vi "Publish Image.vi"(8 "error in (no error)":errorcluster, 9 "Buffer Number":u32, 10 "Image":T1, 11 "Camera in":refnum<class "Camera Actor.lvclass">) -> (0 "error out":errorcluster, 3 "Camera out":refnum<class "Camera Actor.lvclass">)   [LabVIEW 2020, in "Camera Actor.lvlib" / "Camera Actor.lvclass"]
uses:
  Camera Actor.lvclass
  <vilib>/vision/Image Controls.llb/IMAQ Image.ctl
  Camera Actor.lvclass/Camera Actor.ctl
  Camera Actor Messages/New Image Msg/New Image Msg.lvclass/New Image Msg.ctl
  <vilib>/ActorFramework/Message Enqueuer/Message Enqueuer.lvclass/Message Enqueuer.ctl
  <vilib>/ActorFramework/Message Enqueuer/Enqueue.vi
  Camera Actor Messages/New Image Msg/New Image Msg.lvclass
  C:/Program Files (x86)/National Instruments/LabVIEW 2020/vi.lib/ActorFramework/Message/Message.lvclass
  <vilib>/ActorFramework/Message Priority Queue/Priority Enqueue.vi
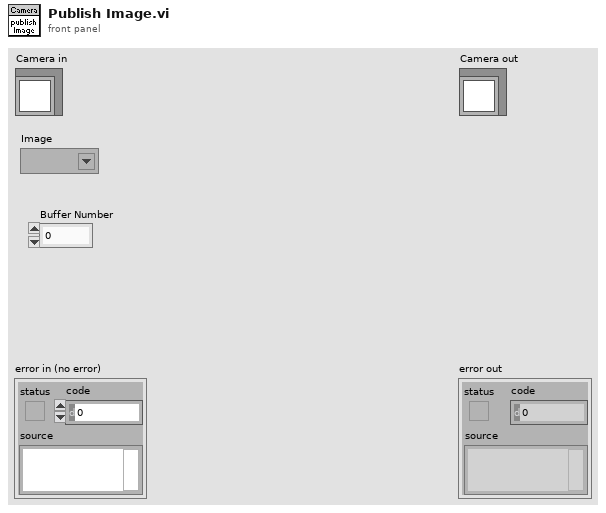
[diagram p1: front panel]
types:
  T1 = typedef "IMAQ Image.ctl" = refnum<image>
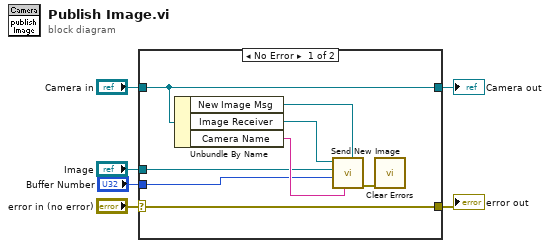
[diagram p0: block diagram]
diagram:
  n1 = case shown="No Error" "error in (no error)" {
    selector: "error in (no error)" -> [w13 w16]
    tunnel: [w13 w16] -> w5
    tunnel: [w12 w15] -> w3
    tunnel: "Camera in" -> [w12 w15]
    tunnel: "Image" -> [w10 _]
    tunnel: "Buffer Number" -> [w9 _]
    frame No Error {
      n2 = Unbundle By Name(w12) -> ("New Image Msg"=w8:refnum<class "New Image Msg.lvclass">, "Image Receiver"=w7:refnum<class "Message Enqueuer.lvclass">, "Camera Name"=w14:string)
      n3 = call "Send New Image.vi"("Message Type"=w8, "Camera"=w14, "Buffer Number"=w9, "Image"=w10, "Message Enqueuer"=w7) -> ("error out"=w11:errorcluster)  [unwired: 5 in, 1 out]
      n4 = call <vilib>:"Clear Errors.vi"("error in (no error)"=w11) -> ()  [unwired: 5 in, 2 out]
    }
    frame Error {
    }
  }
  "error out" <- w5
  "Camera out" <- w3
